vi "LM35_DAQ_Thermostat.vi"() -> ()   [LabVIEW 2019]
uses:
  <vilib>/DAQmx/read.llb/DAQmx Read (Analog DBL 1Chan 1Samp).vi
  <vilib>/DAQmx/miscellaneous.llb/DAQmx Fill In Error Info.vi
panel:
  in  "HISTERESYS [°C]":dbl=2.0 format="%.2f"
  in  "THRESHOLD [°C]":dbl(knob)=22.0 scale=20.0..40.0
  out "ALARM!!!":bool
  out "error out":errorcluster
  in  "stop":bool
  out "Waveform Chart":cluster{dbl, "data":dbl, dbl}(graph)={23.0, "data"=20.974822772540218, 21.0}
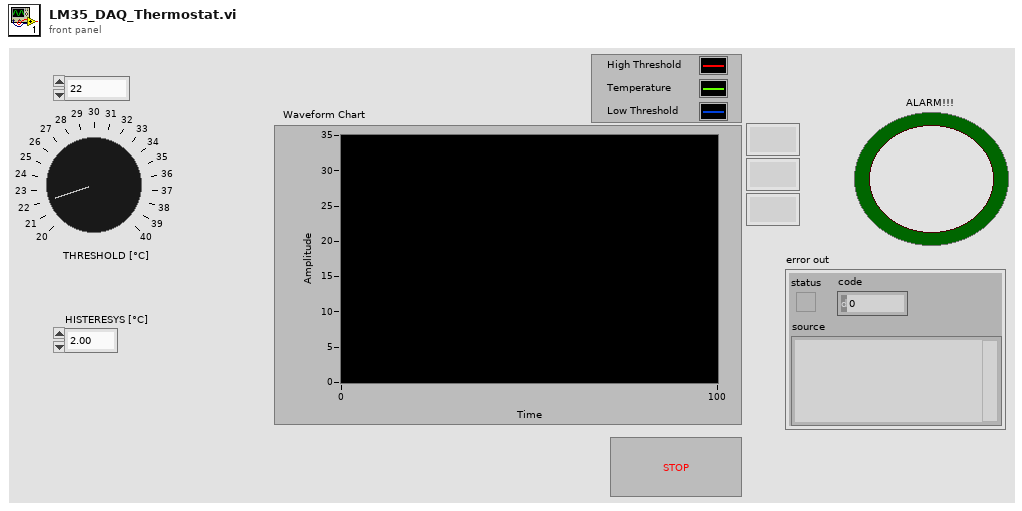
[diagram p1: front panel]
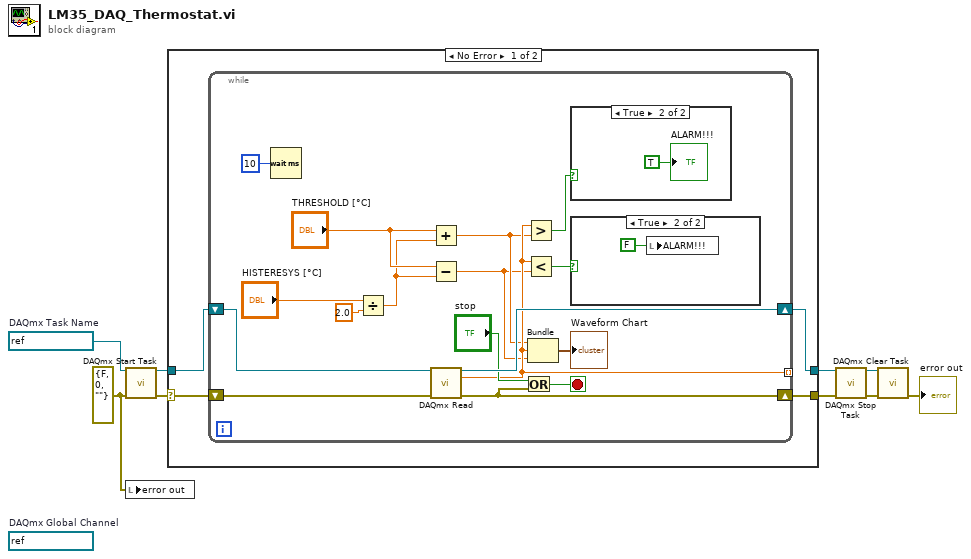
[diagram p0: block diagram]
diagram:
  w2 = refnum<k21> "LM35_Task"  # DAQmx Task Name
  (unwired) refnum<k21> "LM35_GVC"  # DAQmx Global Channel
  w4 = errorcluster {"status"=FALSE, "code"=0, "source"=""} ("error in")
  n1 = call <vilib>:"DAQmx Start Task.vi"("task/channels in"=w2, "error in"=w4) -> ("task out"=w9:refnum<k21>, "error out"=w1:errorcluster)  [unwired: 12 in]
  n2 = local write "error out"(w4) -> ()
  n3 = case shown="No Error" w1 {
    selector: w1 -> [w10 w34]
    tunnel: w9 -> [w13 w33]
    tunnel: [w12 w33] -> w8
    tunnel: [w11 w34] -> w7
    frame No Error {
      n4 = while {
        shift-right: [w28] -> w12
        shift-left: w13 -> [w30]
        shift-right: [w25] -> w11
        shift-left: w10 -> [w29]
        tunnel: [w17] -> _ mode=indexing
        stop <- w26 stop-if-true
        n5 = Wait (ms)(milliseconds to wait=u32 10) -> ()  [unwired: 1 out]
        n6 = Divide(x="HISTERESYS [°C]", y=2.0) -> (x/y=w20:dbl)
        n7 = Add(x="THRESHOLD [°C]", y=w20) -> (x+y=w16:dbl)
        n8 = Subtract(x="THRESHOLD [°C]", y=w20) -> (x-y=w15:dbl)
        n9 = call-poly <vilib>:"DAQmx Read.vi"("task/channels in"=w30, "error in"=w29) -> ("task out"=w28:refnum<k21>, "data"=w17:dbl, "error out"=w25:errorcluster)  [unwired: 11 in]
        n10 = Or(x="stop", y=w25) -> (x .or. y?=w26:bool)
        n11 = Greater?(x=w17, y=w16) -> (0:w19:bool)
        n12 = Less?(x=w17, y=w15) -> (x < y?=w18:bool)
        n13 = Bundle(w16, "data"=w17, w15) -> (→"Waveform Chart":cluster{dbl, "data":dbl, dbl})  [unwired: 1 in]
        n14 = case shown="True" w19 {
          frame False {
          }
          frame True {
            "ALARM!!!" <- TRUE ("SOVRATEMPERATURA!!!")
          }
        }
        n15 = case shown="True" w18 {
          frame False {
          }
          frame True {
            n16 = local write "ALARM!!!"(FALSE ("SOVRATEMPERATURA!!!")) -> ()
          }
        }
      }
    }
    frame Error {
    }
  }
  n17 = call <vilib>:"DAQmx Stop Task.vi"("task/channels in"=w8, "error in"=w7) -> ("task out"=w6:refnum<k21>, "error out"=w5:errorcluster)  [unwired: 12 in]
  n18 = call <vilib>:"DAQmx Clear Task.vi"("task in"=w6, "error in"=w5) -> ("error out"=→"error out":errorcluster)  [unwired: 13 in]
